vi "DAQ Activate Output LINE 0.vi"(5 "error in":errorcluster, 6 "Puerto":dbl, 7 "data":bool) -> (1 "error out":errorcluster, 3 "task out":refnum<k21>)   [LabVIEW 2023]
uses:
  <vilib>/DAQmx/write.llb/DAQmx Write (Digital Bool 1Line 1Point).vi
  <vilib>/DAQmx/miscellaneous.llb/DAQmx Fill In Error Info.vi
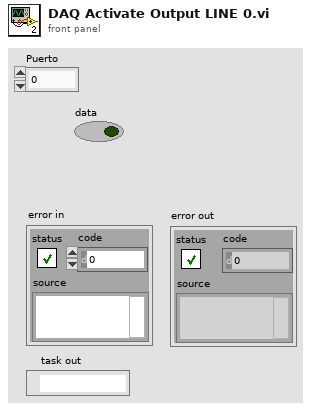
[diagram p1: front panel]
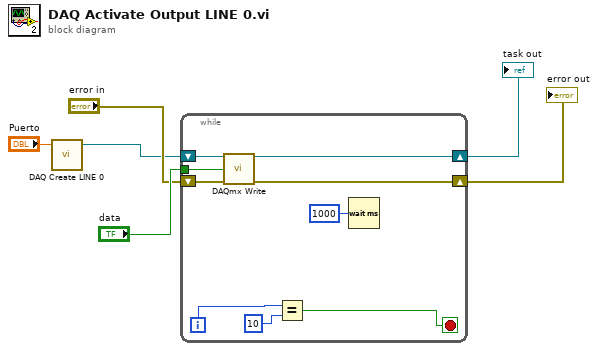
[diagram p0: block diagram]
diagram:
  n1 = call "DAQ Create LINE 0.vi"("Puerto"="Puerto") -> ("task out"=w2:refnum<k21>)  [unwired: 3 in, 1 out]
  n2 = while {
    tunnel: "data" -> [w15]
    shift-right: [w13] -> w4
    shift-left: "error in" -> [w12]
    shift-right: [w14] -> w5
    shift-left: w2 -> [w11]
    i -> [w8]
    stop <- w9 stop-if-true
    n3 = call-poly <vilib>:"DAQmx Write.vi"("task/channels in"=w11, "data"=w15, "error in"=w12) -> ("task out"=w14:refnum<k21>, "error out"=w13:errorcluster)  [unwired: 10 in, 1 out]
    n4 = Equal?(x=w8, y=10) -> (x = y?=w9:bool)
    n5 = Wait (ms)(milliseconds to wait=u32 1000) -> ()  [unwired: 1 out]
  }
  "task out" <- w5
  "error out" <- w4
